vi "Open Library.vi"(8 "error in (no error)":errorcluster, 10 "Full Path":path, 11 "Application in":refnum<vi>) -> (0 "error out":errorcluster, 2 "Library out":refnum<vi>, 3 "Application out":refnum<vi>)   [LabVIEW 2019, in "gRPC Scripting Tools.lvlib"]
uses:
  gRPC Scripting Tools.lvlib
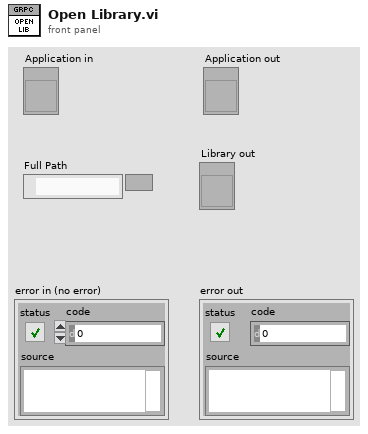
[diagram p1: front panel]
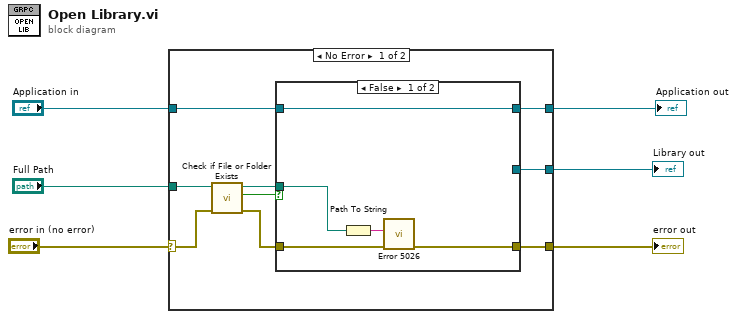
[diagram p0: block diagram]
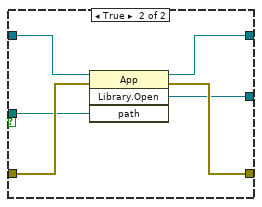
[diagram p2: hidden frame]
diagram:
  n1 = case shown="No Error" "error in (no error)" {
    selector: "error in (no error)" -> [w11 w27]
    tunnel: [w15 w27] -> w6
    tunnel: "Full Path" -> [w10 _]
    tunnel: "Application in" -> [w14 w28]
    tunnel: [w13 _] -> w3
    tunnel: [w12 w28] -> w2
    frame No Error {
      n2 = call <vilib>:"Check if File or Folder Exists.vi"("error in (no error)"=w11, "path"=w10) -> ("error out"=w9:errorcluster, "file or folder exists?"=w8:bool, "dup path"=w7:path)  [unwired: 7 in]
      n3 = case shown="False" w8 {
        tunnel: [w18 w26] -> w15
        tunnel: w14 -> [w20 w25]
        tunnel: [_ w24] -> w13
        tunnel: [w20 w23] -> w12
        tunnel: w9 -> [w19 w22]
        tunnel: w7 -> [w17 w21]
        frame False {
          n4 = Path To String(path=w17) -> (string=w16:string)
          n5 = call "Error 5026.vi"("error in (no error)"=w19, "Library Path"=w16) -> ("error out"=w18:errorcluster)  [unwired: 9 in]
        }
        frame True {
          n6 = invoke class="App" method="Library.Open"(reference=w25, error in=w22, "path"=w21) -> (reference out=w23:refnum<vi>, error out=w26:errorcluster, "Open Library"=w24:refnum<vi>)  [unwired: 1 in, 1 out]
        }
      }
    }
    frame Error {
    }
  }
  "error out" <- w6
  "Library out" <- w3
  "Application out" <- w2
